vi "for_v0_v23.vi"() -> ()   [LabVIEW 2009]
panel:
  out "Waveform Graph":dbl[](graph)=[0.5728905393780532, 0.30340629624240734, 0.5659360583465491, 0.5305907965039671, 0.7676322160112874, 0.23865097144675396, 0.40084710574583626, 0.47939307282891686, 0.22210875222624726, 0.18526860426802783, 0.7586986957161033, 0.7254086278178054, 0.9997247715548976, 0.3896867187317772, 0.2083105101074061, 0.6117164461352309, 0.5770968602206936]
  in  "Numarul de puncte":dbl(slide)=17.441860465116278 scale=0.0..50.0
  in  "stop":bool
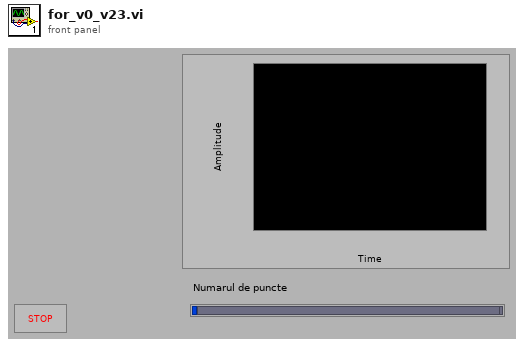
[diagram p1: front panel]
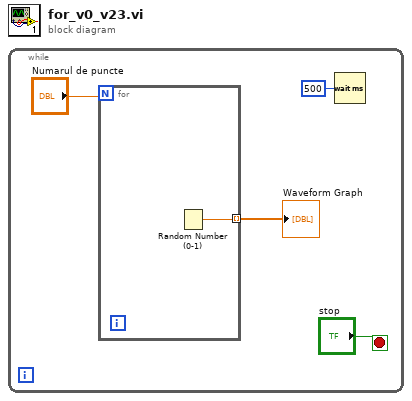
[diagram p0: block diagram]
diagram:
  n1 = while {
    stop <- "stop" stop-if-true
    n2 = for {
      N: "Numarul de puncte" -> [_]
      tunnel: [w5] -> w2 mode=indexing
      n3 = Random Number (0-1)() -> (number: 0 to 1=w5:dbl)
    }
    "Waveform Graph" <- w2
    n4 = Wait (ms)(milliseconds to wait=u32 500) -> ()  [unwired: 1 out]
  }
